vi "Validate Purchase.vi"(8 "error in (no error)":errorcluster, 11 "User Interface in":refnum<class "User Interface.lvclass">) -> (0 "error out":errorcluster, 3 "User Interface out":refnum<class "User Interface.lvclass">)   [LabVIEW 2020, in "User Interface.lvlib" / "User Interface.lvclass"]
uses:
  User Interface.lvclass
  User Interface.lvclass/User Interface.ctl
  <vilib>/ActorFramework/Message Enqueuer/Message Enqueuer.lvclass/Message Enqueuer.ctl
  Dinero Messages/Update Credit Msg/Update Credit Msg.lvclass/Update Credit Msg.ctl
  <vilib>/ActorFramework/Message Enqueuer/Enqueue.vi
  Paquetes Disponibles Messages/Validate Database Msg/Validate Database Msg.lvclass
  C:/Program Files (x86)/National Instruments/LabVIEW 2020/vi.lib/ActorFramework/Message/Message.lvclass
  Dinero Messages/Update Credit Msg/Update Credit Msg.lvclass
  <vilib>/ActorFramework/Message Priority Queue/Priority Enqueue.vi
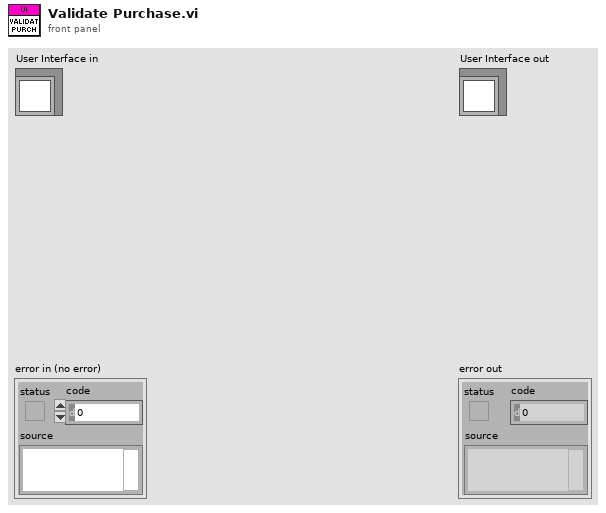
[diagram p1: front panel]
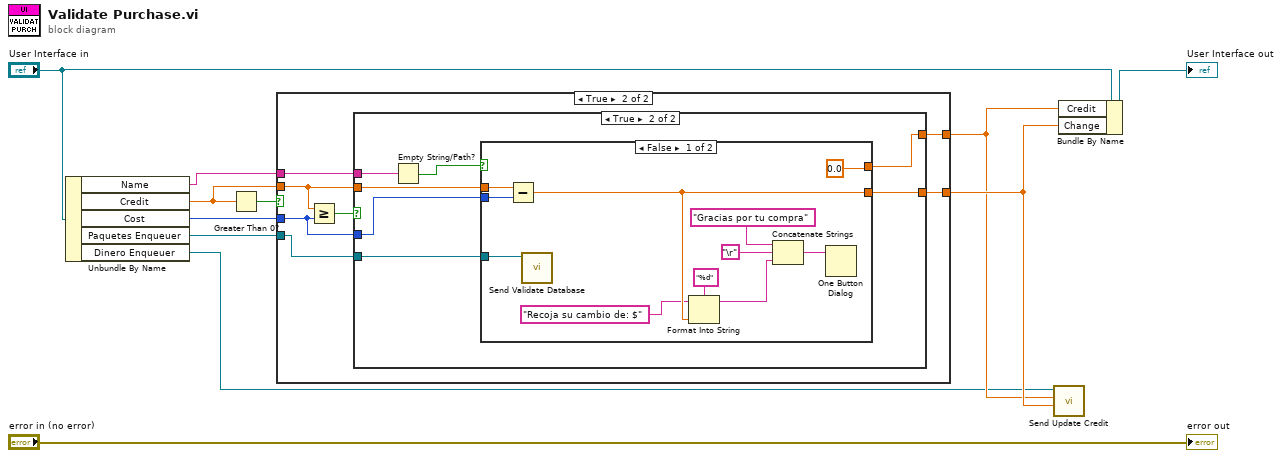
[diagram p0: block diagram]
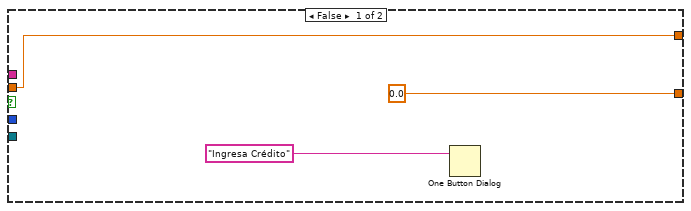
[diagram p2: hidden frame]
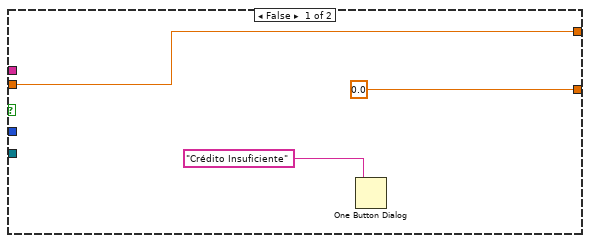
[diagram p3: hidden frame]
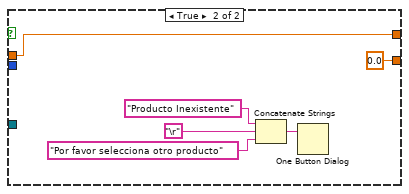
[diagram p4: hidden frame]
diagram:
  n1 = Unbundle By Name("User Interface in") -> ("Name"=w1:string, "Credit"=w7:dbl, "Cost"=w6:u8, "Paquetes Enqueuer"=w2:refnum<class "Message Enqueuer.lvclass">, "Dinero Enqueuer"=w3:refnum<class "Message Enqueuer.lvclass">)
  n2 = Greater Than 0?(x=w7) -> (x > 0?=w8:bool)
  n3 = case shown="True" w8 {
    tunnel: w7 -> [w13 w20]
    tunnel: w6 -> [_ w19]
    tunnel: [0.0 w18] -> w5
    tunnel: [w13 w17] -> w4
    tunnel: w2 -> [_ w16]
    tunnel: w1 -> [_ w15]
    frame False {
      n4 = One Button Dialog(message="Ingresa Crédito") -> ()  [unwired: 1 in, 1 out]
    }
    frame True {
      n5 = Greater Or Equal?(x=w20, y=w19) -> (x >= y?=w21:bool)
      n6 = case shown="True" w21 {
        tunnel: w20 -> [w23 w30]
        tunnel: w19 -> [_ w31]
        tunnel: [0.0 w28] -> w18
        tunnel: [w23 w29] -> w17
        tunnel: w16 -> [_ w27]
        tunnel: w15 -> [_ w26]
        frame False {
          n7 = One Button Dialog(message="Crédito Insuficiente") -> ()  [unwired: 1 in, 1 out]
        }
        frame True {
          n8 = Empty String/Path?(string/path=w26) -> (empty?=w25:bool)
          n9 = case shown="False" w25 {
            tunnel: w31 -> [w42 _]
            tunnel: w30 -> [w41 w44]
            tunnel: [0.0 ("Credit") w44] -> w29
            tunnel: [w36 0.0] -> w28
            tunnel: w27 -> [w32 _]
            frame False {
              n10 = Subtract(x=w41, y=w42) -> (x-y=w36:dbl)
              n11 = call "Send Validate Database.vi"("Message Enqueuer"=w32) -> ()  [unwired: 9 in, 2 out]
              n12 = Format Into String(format string="%d", initial string="Recoja su cambio de: $" ("message"), w36) -> (resulting string=w34:string)  [unwired: 1 in, 1 out]
              n13 = Concatenate Strings("Gracias por tu compra" ("string"), "\r", w34) -> (w38:string)
              n14 = One Button Dialog(message=w38) -> ()  [unwired: 1 in, 1 out]
            }
            frame True {
              n15 = Concatenate Strings("Producto Inexistente" ("message"), "\r", "Por favor selecciona otro producto" ("string")) -> (w45:string)
              n16 = One Button Dialog(message=w45) -> ()  [unwired: 1 in, 1 out]
            }
          }
        }
      }
    }
  }
  n17 = call "Send Update Credit.vi"("Change"=w5, "Credit"=w4, "Message Enqueuer"=w3) -> ()  [unwired: 7 in, 2 out]
  n18 = Bundle By Name(cluster="User Interface in", "Credit"=w4, "Change"=w5) -> (→"User Interface out":refnum<class "User Interface.lvclass">)
  "error out" <- "error in (no error)"
